vi "Validate Choice.vi"(8 "error in (no error)":errorcluster, 10 "Choice":T1, 11 "Reversi in":refnum<class "Reversi.lvclass">) -> (0 "error out":errorcluster, 3 "Reversi out":refnum<class "Reversi.lvclass">)   [LabVIEW 2020, in "Reversi.lvlib" / "Reversi.lvclass"]
uses:
  Reversi.lvclass
  Space Cluster.ctl
  Space Coordinates.ctl
  Space Ring.ctl
  Reversi.lvclass/Reversi.ctl
  Human/Human.lvclass
  C:/dev/SoL/sol-reversi/ProjectTemplates/Source/SummerOfLabVIEW/Reversi/template/Reversi/Player/Player.lvclass
  C:/dev/SoL/sol-reversi/ProjectTemplates/Source/SummerOfLabVIEW/Reversi/template/Reversi/Human/Human.lvclass
  Player/Player.lvclass
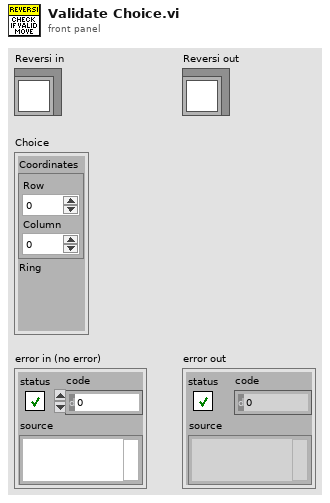
[diagram p1: front panel]
types:
  T1 = typedef "Reversi.lvlib/Reversi.lvclass/Space Cluster.ctl" = cluster{"Coordinates":T2, "Ring":T3}
  T2 = typedef "Reversi.lvlib/Reversi.lvclass/Space Coordinates.ctl" = cluster{"Row":i32, "Column":i32}
  T3 = typedef "Reversi.lvlib/Reversi.lvclass/Space Ring.ctl" = u16
  T4 = typedef "Reversi.lvlib/Reversi.lvclass/Turn Enum.ctl" = enum16{"Black", "White"}
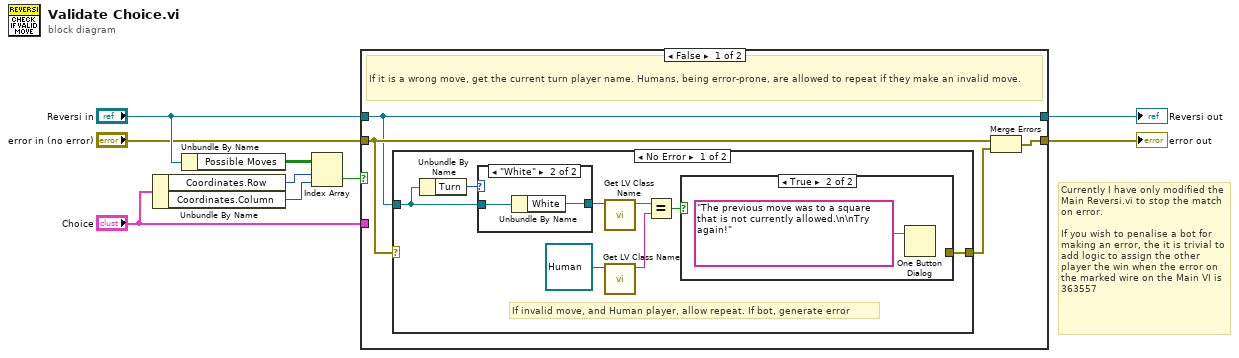
[diagram p0: block diagram]
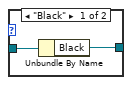
[diagram p2: hidden frame]
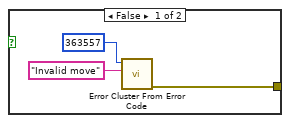
[diagram p3: hidden frame]
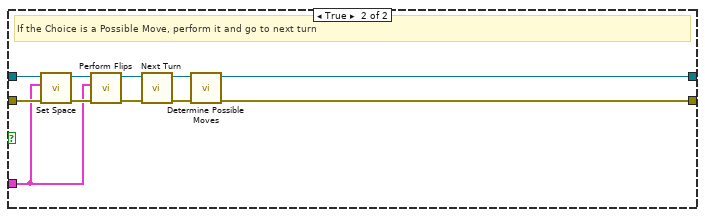
[diagram p5: hidden frame]
diagram:
  # "Currently I have only modified the Main Reversi.vi to stop the match on error.\n\nIf you wish to penalise a bot for making an error, the it is trivial to add logic to assign the other player the win when the error on the marked wire on the Main VI is 363557"
  n1 = Unbundle By Name("Choice") -> ("Coordinates.Row"=w7:i32, "Coordinates.Column"=w6:i32)
  n2 = Unbundle By Name("Reversi in") -> ("Possible Moves"=w8:bool[][])
  n3 = Index Array(array=w8, index (row)=w7, index (col)=w6) -> (element=w5:bool)
  n4 = case shown="False" w5 {
    tunnel: [w12 w31] -> w1
    tunnel: "Reversi in" -> [w12 w41]
    tunnel: "error in (no error)" -> [w13 w40]
    tunnel: [w10 w33] -> w2
    tunnel: "Choice" -> [_ w37]
    frame False {
      # "If it is a wrong move, get the current turn player name. Humans, being error-prone, are allowed to repeat if they make an invalid move."
      n5 = case shown="No Error" w13 {
        selector: w13 -> [_ w30]
        tunnel: w12 -> [w18 _]
        tunnel: [w16 w30] -> w11
        frame No Error {
          # "If invalid move, and Human player, allow repeat. If bot, generate error"
          n6 = Unbundle By Name(w18) -> ("Turn"=w19:T4)
          n7 = case shown="\"White\"" w19 {
            tunnel: w18 -> [w23 w25]
            tunnel: [w22 w24] -> w17
            frame "Black" {
              n8 = Unbundle By Name(w23) -> ("Black"=w22:refnum<class "Player.lvclass">)
            }
            frame "White" {
              n9 = Unbundle By Name(w25) -> ("White"=w24:refnum<class "Player.lvclass">)
            }
          }
          n10 = call <vilib>:"Get LV Class Name.vi"("object"=w17) -> ("class name"=w21:string)  [unwired: 9 in, 1 out]
          n11 = call <vilib>:"Get LV Class Name.vi"("object"=refnum<class "Human.lvclass"> refnum ("Reversi.lvlib:Human.lvclass")) -> ("class name"=w14:string)  [unwired: 9 in, 1 out]
          n12 = Equal?(x=w21, y=w14) -> (x = y?=w20:bool)
          n13 = case shown="True" w20 {
            tunnel: [w28 _] -> w16
            frame False {
              # "Bot players making errors are frowned upon"
              n14 = call <vilib>:"Error Cluster From Error Code.vi"("error message (\"\")"="Invalid move" ("error message (\"\")"), "error code (0)"=363557) -> ("error out"=w28:errorcluster)  [unwired: 7 in]
            }
            frame True {
              # "Human is told the move was invalid and allowed to repeat the turn"
              n15 = One Button Dialog(message="The previous move was to a square that is not currently allowed.\n\nTry again!") -> ()  [unwired: 1 in, 1 out]
            }
          }
        }
        frame Error {
          # "Only Errors possible are 9998 or 9999 right now. Just pass the error through. This ensures the Illegal Move made dialog is not popped up for the Human player"
        }
      }
      n16 = Merge Errors(w13, w11) -> (w10:errorcluster)
    }
    frame True {
      # "If the Choice is a Possible Move, perform it and go to next turn"
      n17 = call "Set Space.vi"("error in (no error)"=w40, "Space"=w37, "Reversi in"=w41) -> ("error out"=w38:errorcluster, "Reversi out"=w39:refnum<class "Reversi.lvclass">)  [unwired: 7 in]
      n18 = call "Perform Flips.vi"("error in (no error)"=w38, "Choice"=w37, "Reversi in"=w39) -> ("error out"=w36:errorcluster, "Reversi out"=w34:refnum<class "Reversi.lvclass">)  [unwired: 7 in]
      n19 = call "Next Turn.vi"("error in (no error)"=w36, "Reversi in"=w34) -> ("error out"=w35:errorcluster, "Reversi out"=w32:refnum<class "Reversi.lvclass">)  [unwired: 8 in]
      n20 = call "Determine Possible Moves.vi"("error in (no error)"=w35, "Reversi in"=w32) -> ("error out"=w33:errorcluster, "Reversi out"=w31:refnum<class "Reversi.lvclass">)  [unwired: 8 in]
    }
  }
  "error out" <- w2
  "Reversi out" <- w1
